vi "Detector Send New Image Message.vi"(8 "error in (no error)":errorcluster, 11 "New Images":T2[](array[typedef])) -> (0 "error out":errorcluster, 3 "Image Messages":T1[](array[typedef]) {"Detector #" items=["None", "YJ", "HK"]})   [LabVIEW 2024]
uses:
  Detector Image typedef cluster.ctl
  Subsystems/SS cluster New Image Data.ctl
  Detector Class.lvclass
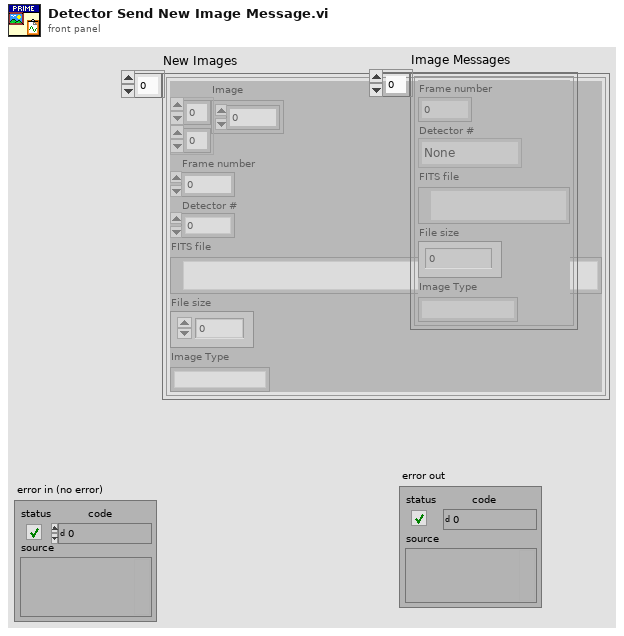
[diagram p1: front panel]
types:
  T1 = typedef "SS cluster New Image Data.ctl" = cluster{"Frame number":i32, "Detector #":u16, "FITS file":path, "File size":i64, "Image Type":string}
  T2 = typedef "Detector Class.lvclass/Detector Image typedef cluster.ctl" = cluster{"Image":sgl[][], "Frame number":i32, "Detector #":u16, "FITS file":path, "File size":i64, "Image Type":string}
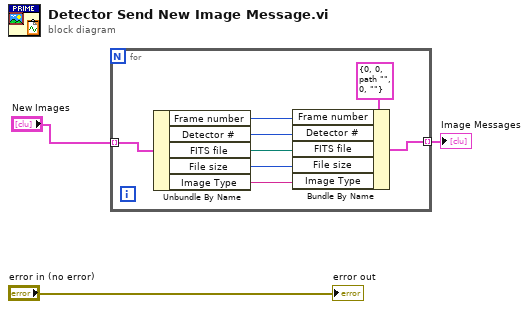
[diagram p0: block diagram]
diagram:
  n1 = for {
    tunnel: "New Images" -> [w6] mode=indexing
    tunnel: [w5] -> w1 mode=indexing
    n2 = Unbundle By Name(w6) -> ("Frame number"=w10:i32, "Detector #"=w9:u16, "FITS file"=w8:path, "File size"=w7:i64, "Image Type"=w4:string)
    n3 = Bundle By Name(cluster=T1 {"Frame number"=0, "Detector #"=0, "FITS file"=path "", "File size"=0, "Image Type"=""} ("New Image"), "Frame number"=w10, "Detector #"=w9, "FITS file"=w8, "File size"=w7, "Image Type"=w4) -> (w5:T1)
  }
  "Image Messages" <- w1
  "error out" <- "error in (no error)"
